vi "registerRunEvents.vi"(8 "error in (no error)":errorcluster, 11 "ExperimentControlEvents in":refnum<class "ExperimentControlEvents.lvclass">) -> (0 "error out":errorcluster, 3 "ExperimentControlEvents out":refnum<class "ExperimentControlEvents.lvclass">)   [LabVIEW 2009, in "Views.lvlib" / "ExperimentControl.lvlib" / "ExperimentControlEvents.lvclass"]
uses:
  ExperimentControlEvents.lvclass
  Events/Event.lvclass
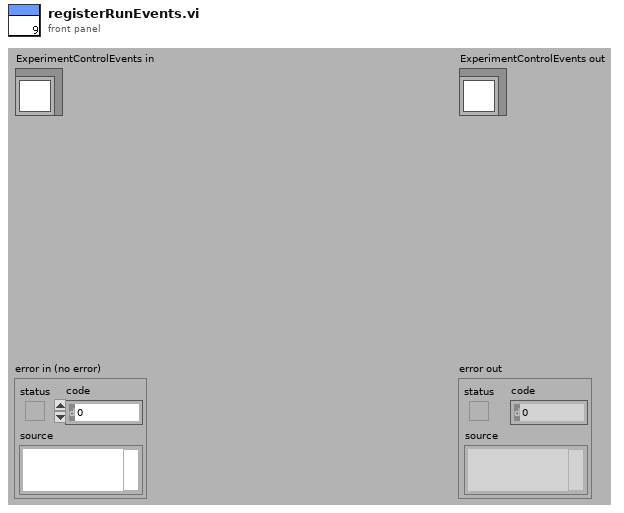
[diagram p1: front panel]
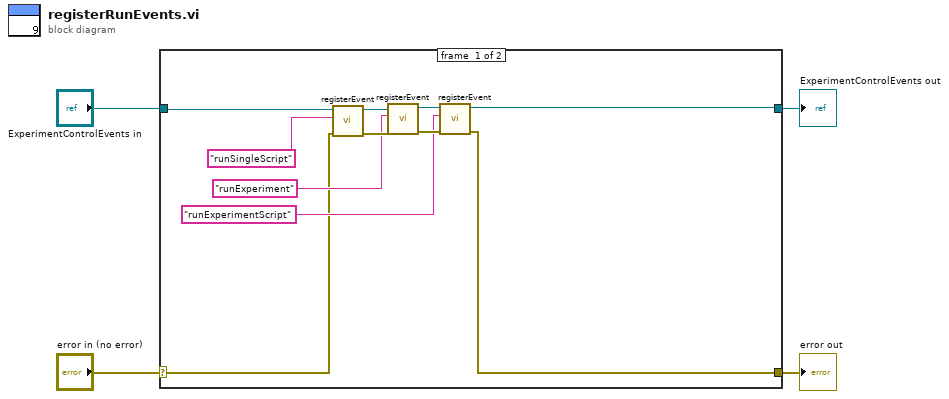
[diagram p0: block diagram]
diagram:
  n1 = case shown="No Error" "error in (no error)" {
    selector: "error in (no error)" -> [w6 w17]
    tunnel: [w5 w17] -> w3
    tunnel: [w9 w16] -> w1
    tunnel: "ExperimentControlEvents in" -> [w15 w16]
    frame #0 {
      n2 = call "registerEvent.vi"("error in (no error)"=w6, "name"="runSingleScript", "Event in"=w15) -> ("error out"=w12:errorcluster, "Event out"=w13:refnum<class "ExperimentControlEvents.lvclass">)  [unwired: 7 in]
      n3 = call "registerEvent.vi"("error in (no error)"=w12, "name"="runExperiment", "Event in"=w13) -> ("error out"=w10:errorcluster, "Event out"=w11:refnum<class "ExperimentControlEvents.lvclass">)  [unwired: 7 in]
      n4 = call "registerEvent.vi"("error in (no error)"=w10, "name"="runExperimentScript", "Event in"=w11) -> ("error out"=w5:errorcluster, "Event out"=w9:refnum<class "ExperimentControlEvents.lvclass">)  [unwired: 7 in]
    }
    frame #1 {
    }
  }
  "error out" <- w3
  "ExperimentControlEvents out" <- w1
